vi "get init random.vi"(8 "error in (no error)":errorcluster, 10 "init_random":T1, 11 "id":i32) -> (0 "error out":errorcluster, 2 "init_random out":T1, 3 "function return":i32)   [LabVIEW 2012, in "libximc.lvlib"]
doc: "result_t XIMC_API get_init_random (device_t id, init_random_t* init_random);"
uses:
  libximc.lvlib
  libximc.dll
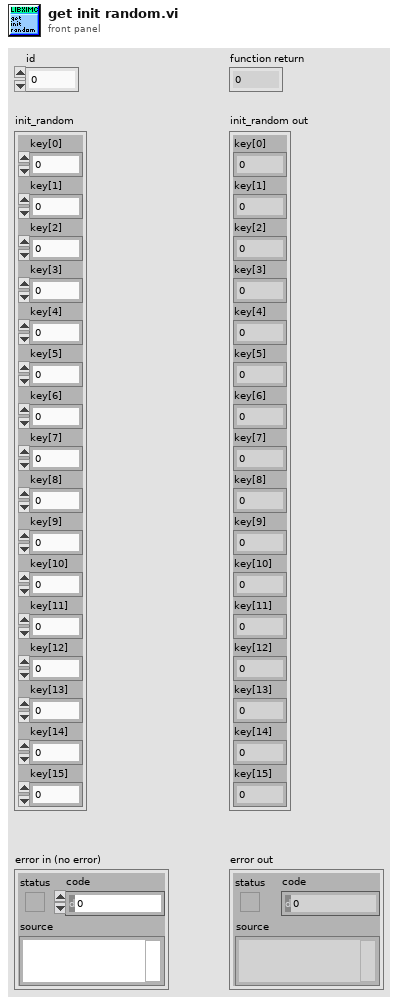
[diagram p1: front panel]
types:
  T1 = cluster{"key[0]":u8, "key[1]":u8, "key[2]":u8, "key[3]":u8, "key[4]":u8, "key[5]":u8, "key[6]":u8, "key[7]":u8, "key[8]":u8, "key[9]":u8, "key[10]":u8, "key[11]":u8, "key[12]":u8, "key[13]":u8, "key[14]":u8, "key[15]":u8}
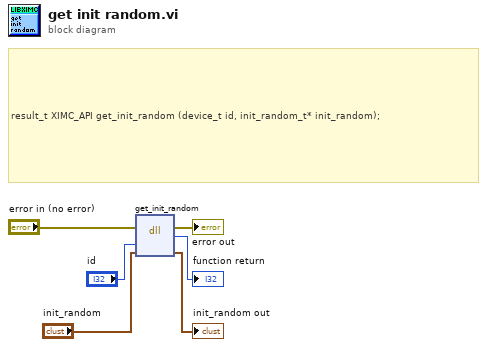
[diagram p0: block diagram]
diagram:
  # "result_t XIMC_API get_init_random (device_t id, init_random_t* init_random);"
  n1 = dll-call lib="C:/Users/Vasily/Att_examples/LabVIEW_example/libximc.*" fn="get_init_random"(error in="error in (no error)", "id"="id", "init_random"="init_random") -> (error out=→"error out":errorcluster, →"function return":i32, "init_random"=→"init_random out":T1)  [unwired: 3 in, 1 out]
